vi "GEA2 Serial Get Source Address.vi"(8 "Error In":errorcluster, 9 "Current Read Index":i32, 10 "ReadArray":u8[](array[numeric]), 11 "CRCArray":u8[](array[numeric])) -> (0 "Error Out":errorcluster, 1 "Source Address":u8, 2 "Current Read Index":i32, 3 "CRC Array":u8[](array[numeric]))   [LabVIEW 2014]
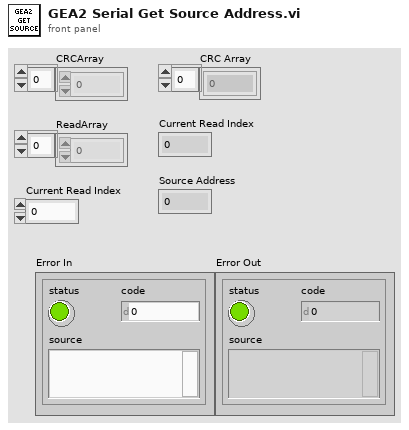
[diagram p1: front panel]
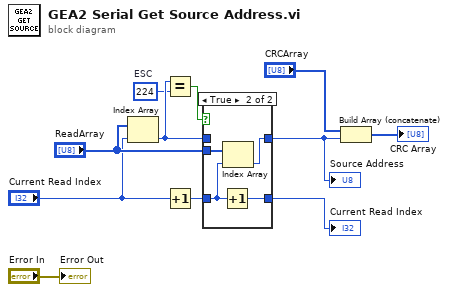
[diagram p0: block diagram]
diagram:
  w2 = u8 224  # ESC
  n1 = Index Array(array="ReadArray", index="Current Read Index") -> (element=w7:u8)
  n2 = Equal?(x=w7, y=w2) -> (x = y?=w3:bool)
  n3 = Increment(x="Current Read Index") -> (x+1=w9:i32)
  n4 = case shown="True" w3 {
    tunnel: [w13 w16] -> w11
    tunnel: [w12 w14] -> w10
    tunnel: "ReadArray" -> [_ w17]
    tunnel: w7 -> [w13 _]
    tunnel: w9 -> [w12 w15]
    frame False {
    }
    frame True {
      n5 = Increment(x=w15) -> (x+1=w14:i32)
      n6 = Index Array(array=w17, index=w15) -> (element=w16:u8)
    }
  }
  "Source Address" <- w11
  "Current Read Index" <- w10
  n7 = Build Array (concatenate)("CRCArray", w11) -> (→"CRC Array":u8[])
  "Error Out" <- "Error In"
